vi "Measure Temperature Query.vi"(0 "VISA resource name":refnum<visa-resource-name>, 11 "error in (no error)":errorcluster) -> (4 "VISA resource name out":refnum<visa-resource-name>, 6 "write return count":u32, 8 "read return count":u32, 10 "read buffer":string, 15 "error out":errorcluster)   [LabVIEW 2023, in "ACM Visa Driver.lvlib"]
uses:
  ACM Visa Driver.lvlib
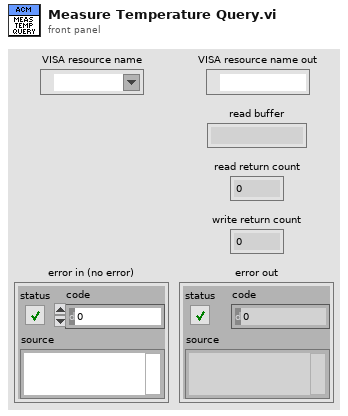
[diagram p1: front panel]
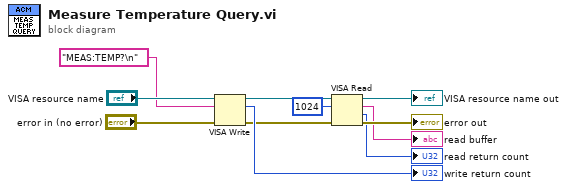
[diagram p0: block diagram]
diagram:
  n1 = VISA Write(VISA resource name="VISA resource name", write buffer="MEAS:TEMP?\n", error in (no error)="error in (no error)") -> (VISA resource name out=w5:refnum<visa-resource-name>, return count=→"write return count":u32, error out=w7:errorcluster)
  n2 = VISA Read(VISA resource name=w5, byte count=u32 1024, error in (no error)=w7) -> (VISA resource name out=→"VISA resource name out":refnum<visa-resource-name>, read buffer=→"read buffer":string, return count=→"read return count":u32, error out=→"error out":errorcluster)
